vi "判定取舍1.vi"(1 "输入表格":string[][](table)) -> (0 "输出表格":string[][](table))   [LabVIEW 2017]
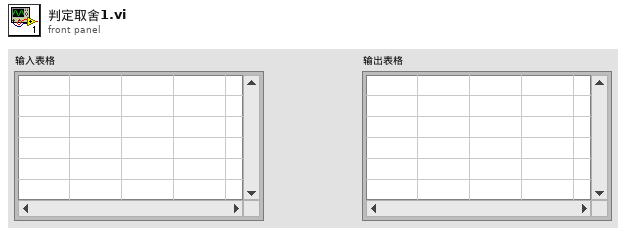
[diagram p1: front panel]
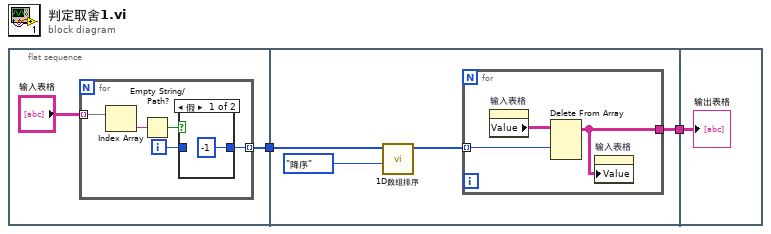
[diagram p0: block diagram]
diagram:
  n1 = flat-sequence {
    tunnel: [w4] -> w2
    tunnel: w2 -> [w14]
    tunnel: [w15] -> w1
    tunnel: w1 -> [w19]
    frame #0 {
      n2 = for {
        tunnel: "输入表格" -> [w9] mode=indexing
        tunnel: [w7] -> w4 mode=indexing
        i -> [w8]
        n3 = Index Array(array=w9) -> (element=w6:string)  [unwired: 1 in]
        n4 = Empty String/Path?(string/path=w6) -> (empty?=w5:bool)
        n5 = case shown="假" w5 {
          tunnel: w8 -> [_ w11]
          tunnel: [-1 w11] -> w7
          frame False {
          }
          frame True {
          }
        }
      }
    }
    frame #1 {
      n6 = call-poly "1D数组排序.vi"("升降序"=enum16{"升序", "降序"}."降序", "输入数组"=w14) -> ("排序后数组"=w12:i32[])  [unwired: 7 in, 2 out]
      n7 = for {
        tunnel: w12 -> [w18] mode=indexing
        tunnel: [w16] -> w15
        n8 = property on="输入表格" class="Tbl (严格)"() -> ("Value"=w17:string[][])  [unwired: 2 in, 2 out]
        n9 = Delete From Array(array=w17, index (row)=w18) -> (array with subset deleted=w16:string[][])  [unwired: 2 in, 1 out]
        n10 = property on="输入表格" class="Tbl (严格)"("Value"=w16) -> ()  [unwired: 2 in, 2 out]
      }
    }
    frame #2 {
      "输出表格" <- w19
    }
  }
